vi "Property Tree_Build Tree_RW.vi"(5 "Tree Type":enum16{"Main", "Write", "Read"}(ring), 7 "Action":T3, 8 "error in":errorcluster, 9 "Displayed Items":string[](array[string]), 10 "Properties for Tree":T2(array[cluster]), 11 "Tree Ref":refnum<vi>) -> (0 "error out":errorcluster, 3 "Tree Ref Out":refnum<vi>, 4 "exe time (ms)":u32)   [LabVIEW 2023]
doc: "Build R/W trees based on displayed items in main tree. This is done bc the open/close items properties don't apply to the R/W trees, who have all items set to indent=0 so symbols can be displayed."
uses:
  controls/action enum.ctl
panel:
  out "Tree Arr":T1(array[cluster])
  in  "Tree":string[](tree)
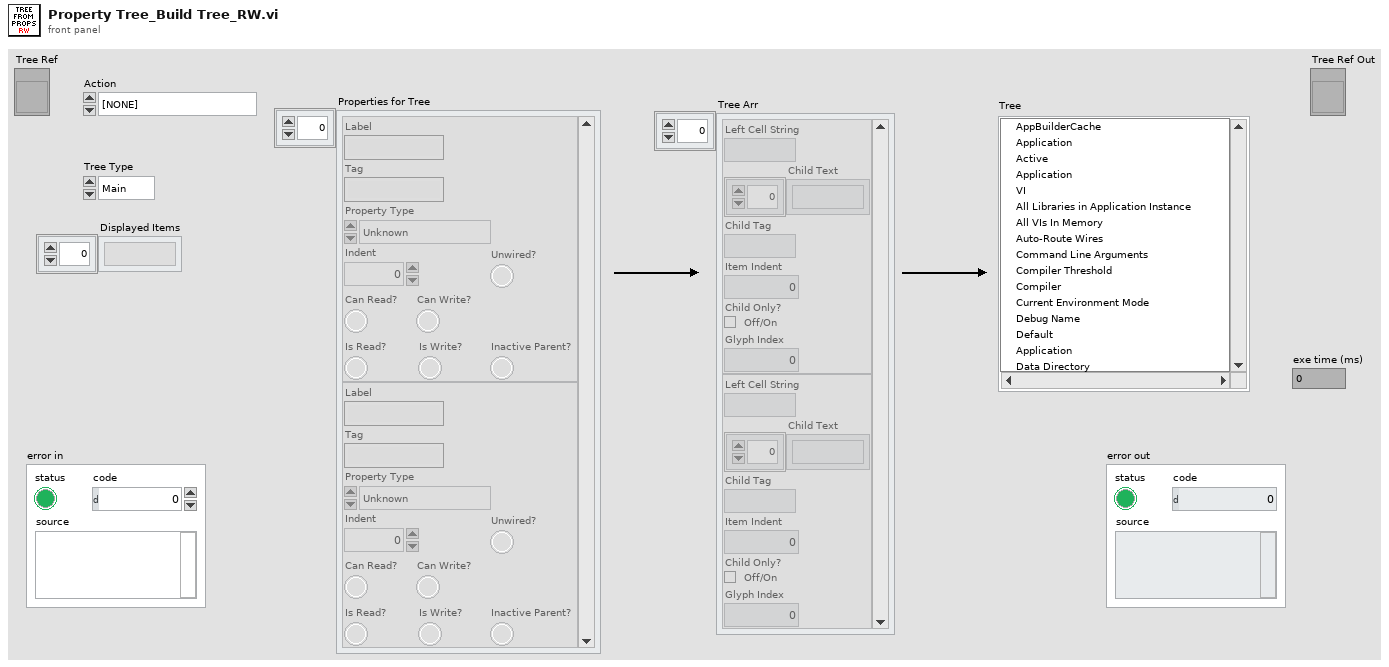
[diagram p1: front panel]
types:
  T1 = cluster{"Left Cell String":string, "Child Text":string[], "Child Tag":string, "Item Indent":i32, "Child Only?":bool, "Glyph Index":i32}[]
  T2 = cluster{"Label":string, "Tag":string, "Property Type":enum16{"Unknown", "Base", "Scripting", "Private", "Deprecated", "None", "Divider"}, "Indent":u16, "Can Read?":bool, "Can Write?":bool, "Is Read?":bool, "Is Write?":bool, "Inactive Parent?":bool, "Unwired?":bool}[]
  T3 = typedef "action enum.ctl" = enum16{"[NONE]", "Wire Bundle", "Wire Unbundle", "Terminal Unbundle", "Terminal Bundle", "Bundler Move Up", "Bundler Move Down", "Bundler Insert", "Bundler Remove", "Bundler Remove Unwired", "Bundler Rearrange", "In Place Insert", "In Place Remove", "In Place Remove Unwired", "In Place Rearrange", "Wire Properties", "Wire Method", "Terminal Properties", "Terminal Method", "Property Move Up", "Property Move Down", "Properties Insert", "Properties Remove", "Properties Remove Unwired", "Properties Rearrange", "Method Change", "Class for Constant", "Class For Control", "Class For Node", "Class Name to Clipboard"}
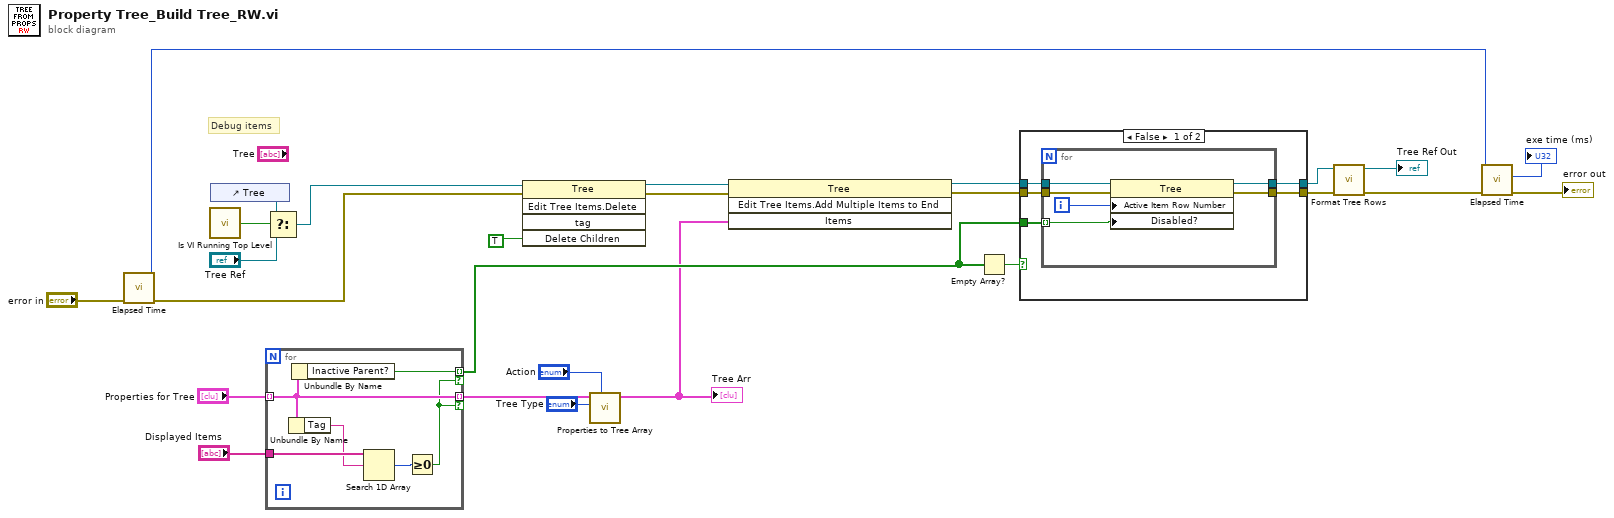
[diagram p0: block diagram]
diagram:
  # "Debug items"
  n1 = call "Elapsed Time.vi"("error in"="error in") -> ("error out"=w13:errorcluster, "millisecond timer value"=w12:u32)  [unwired: 7 in, 2 out]
  n2 = call "Is VI Running Top Level.vi"() -> ("Top Level?"=w25:bool)  [unwired: 5 in]
  n3 = control-ref of="Tree"() -> (w23:refnum<vi>)
  n4 = for {
    tunnel: "Properties for Tree" -> [w29] mode=indexing
    tunnel: "Displayed Items" -> [w32]
    tunnel: [w29] -> w5 mode=indexing if=w27
    tunnel: [w28] -> w9 mode=indexing if=w27
    n5 = Unbundle By Name(w29) -> ("Tag"=w31:string)
    n6 = Unbundle By Name(w29) -> ("Inactive Parent?"=w28:bool)
    n7 = Search 1D Array(1D array=w32, element=w31) -> (index of element=w30:i32)  [unwired: 1 in]
    n8 = Greater Or Equal To 0?(x=w30) -> (x >= 0?=w27:bool)
  }
  n9 = Select(t=w23, s=w25, f="Tree Ref") -> (s? t:f=w22:refnum<vi>)
  n10 = invoke class="Tree" method="Edit Tree Items.Delete"(reference=w22, error in=w13, "Delete Children"=TRUE ("Delete Children?")) -> (reference out=w18:refnum<vi>, error out=w17:errorcluster)  [unwired: 2 in, 3 out]
  n11 = call "Properties to Tree Array.vi"("Action"="Action", "Tree Type"="Tree Type", "Properties for Tree"=w5) -> ("Tree Arr"=w7:T1)  [unwired: 8 in]
  "Tree Arr" <- w7
  n12 = invoke class="Tree" method="Edit Tree Items.Add Multiple Items to End"(reference=w18, error in=w17, "Items"=w7) -> (reference out=w20:refnum<vi>, error out=w19:errorcluster)  [unwired: 1 in, 2 out]
  n13 = Empty Array?(array=w9) -> (empty?=w21:bool)
  n14 = case shown="False" w21 {
    tunnel: w20 -> [w37 w45]
    tunnel: [w36 w45] -> w3
    tunnel: w19 -> [w35 w44]
    tunnel: [w34 w44] -> w4
    tunnel: w9 -> [w33 _]
    frame False {
      n15 = for {
        tunnel: w37 -> [w43]
        tunnel: [w41] -> w36
        tunnel: w35 -> [w40]
        tunnel: [w39] -> w34
        tunnel: w33 -> [w38] mode=indexing
        i -> [w42]
        n16 = property class="Tree"(reference=w43, error in=w40, "Active Item Row Number"=w42, "Disabled?"=w38) -> (reference out=w41:refnum<vi>, error out=w39:errorcluster)
      }
    }
    frame True {
    }
  }
  n17 = call "Format Tree Rows.vi"("error in"=w4, "Tree Ref"=w3) -> ("error out"=w1:errorcluster, "Tree Ref out"=→"Tree Ref Out":refnum<vi>)  [unwired: 8 in]
  n18 = call "Elapsed Time.vi"("error in"=w1, "past time"=w12) -> ("error out"=→"error out":errorcluster, "elapsed time (ms)"=→"exe time (ms)":u32)  [unwired: 6 in, 2 out]
